vi "T_sat_correlation.vi"(0 "P [Pa]":dbl) -> (1 "T Sat [C]":dbl, 2 "T Sat [K]":dbl)   [LabVIEW 2015]
uses:
  <vilib>/express/express arith-compare/Formula/XNode/ExpressFormulaBlockNode.xnode
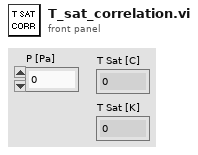
[diagram p1: front panel]
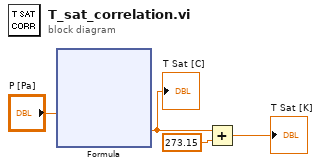
[diagram p0: block diagram]
diagram:
  n1 = xnode "Formula"("P"="P [Pa]") -> ("Result"=w2:dbl)  [unwired: 1 in, 1 out]
  "T Sat [C]" <- w2
  n2 = Add(x=w2, y=273.15) -> (x+y=→"T Sat [K]":dbl)
